vi "WriteLog.vi"(9 "relative seconds in":dbl, 10 "Numeric":i32, 11 "Byte Stream File in":refnum<file>) -> (2 "x-y":dbl, 3 "relative seconds out":dbl)   [LabVIEW 2016]
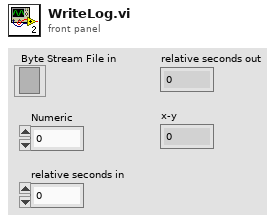
[diagram p1: front panel]
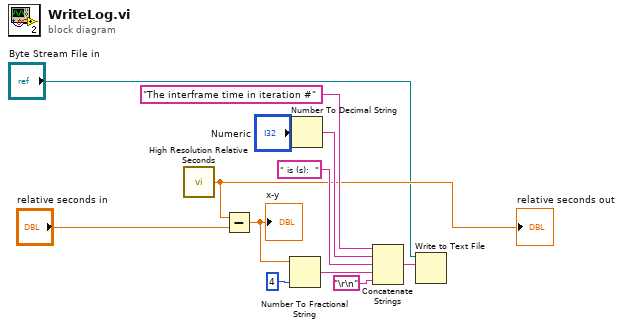
[diagram p0: block diagram]
diagram:
  n1 = call <vilib>:"High Resolution Relative Seconds.vi"() -> ("relative seconds"=w3:dbl)
  "relative seconds out" <- w3
  n2 = Subtract(x=w3, y="relative seconds in") -> (x-y=w5:dbl)
  "x-y" <- w5
  n3 = Number To Fractional String(number=w5, precision (6)=i16 4 ("width (-)")) -> (F-format string=w8:string)  [unwired: 2 in]
  n4 = Number To Decimal String(number="Numeric") -> (decimal integer string=w10:string)  [unwired: 1 in]
  n5 = Concatenate Strings("The interframe time in iteration #" ("string"), w10, " is (s):  " ("string"), w8, "\r\n") -> (w1:string)
  n6 = Write to Text File(file (use dialog)="Byte Stream File in", text=w1) -> ()  [unwired: 2 in, 3 out]
